vi "Create.vi"(8 "error in (no error)":errorcluster) -> (0 "error out":errorcluster, 3 "Error Result out":refnum<class "Error Result.lvclass">)   [LabVIEW 2020, in "Promises.lvlib" / "Error Result.lvclass"]
uses:
  Error Result.lvclass
  Error Result.lvclass/Error Result.ctl
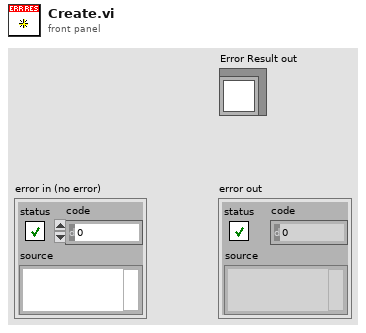
[diagram p1: front panel]
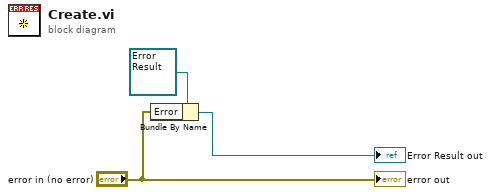
[diagram p0: block diagram]
diagram:
  n1 = Bundle By Name(cluster=refnum<class "Error Result.lvclass"> refnum ("Error Result in"), "Error"="error in (no error)") -> (→"Error Result out":refnum<class "Error Result.lvclass">)
  "error out" <- "error in (no error)"
